vi "Do Zig Zag.vi"(9 "Wall Left?":bool=TRUE) -> (1 "Target Angle":dbl=1.5707963267948966)   [LabVIEW 2017]
uses:
  Globals/Zig Zag Global.vi
  Globals/Pose.vi
panel:
  in  "Forward Distance":dbl=200.0
  in  "Current Point":i32=4
  out "Initial Encoder Position":cluster{"X":dbl, "Y":dbl}={"X"=3425.411384902823, "Y"=-4669.166577156122}
  out "Initial Wall Distance":dbl=209.0
  out "Initial Wall Angle":dbl=1.5707963267948966
  in  "Target Angles&X Points":T1(array[cluster])=[{"Target Angle"=0.7, "Target X Point"=200.0}, {"Target Angle"=-0.7, "Target X Point"=280.0}, {"Target Angle"=0.5, "Target X Point"=250.0}]
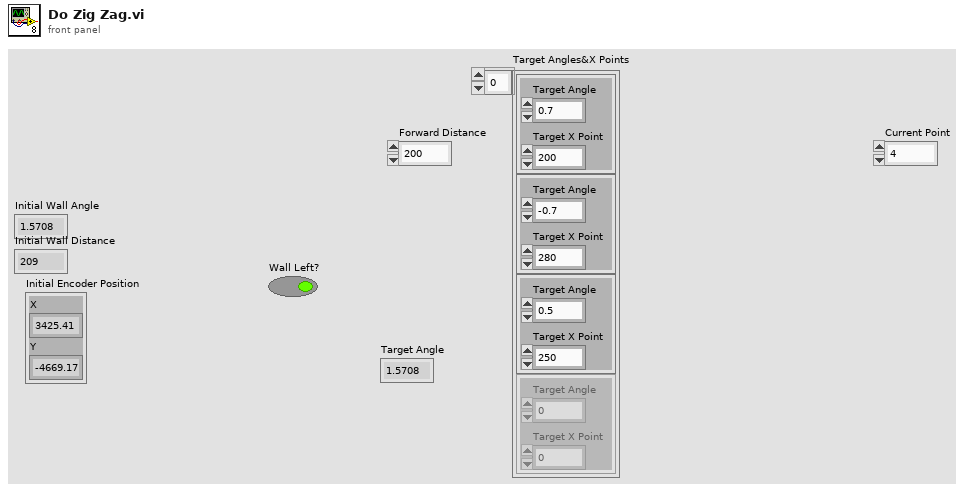
[diagram p1: front panel]
types:
  T1 = cluster{"Target Angle":dbl, "Target X Point":dbl}[]
  T2 = cluster{"Target Angle":dbl, "Target X Point":dbl}
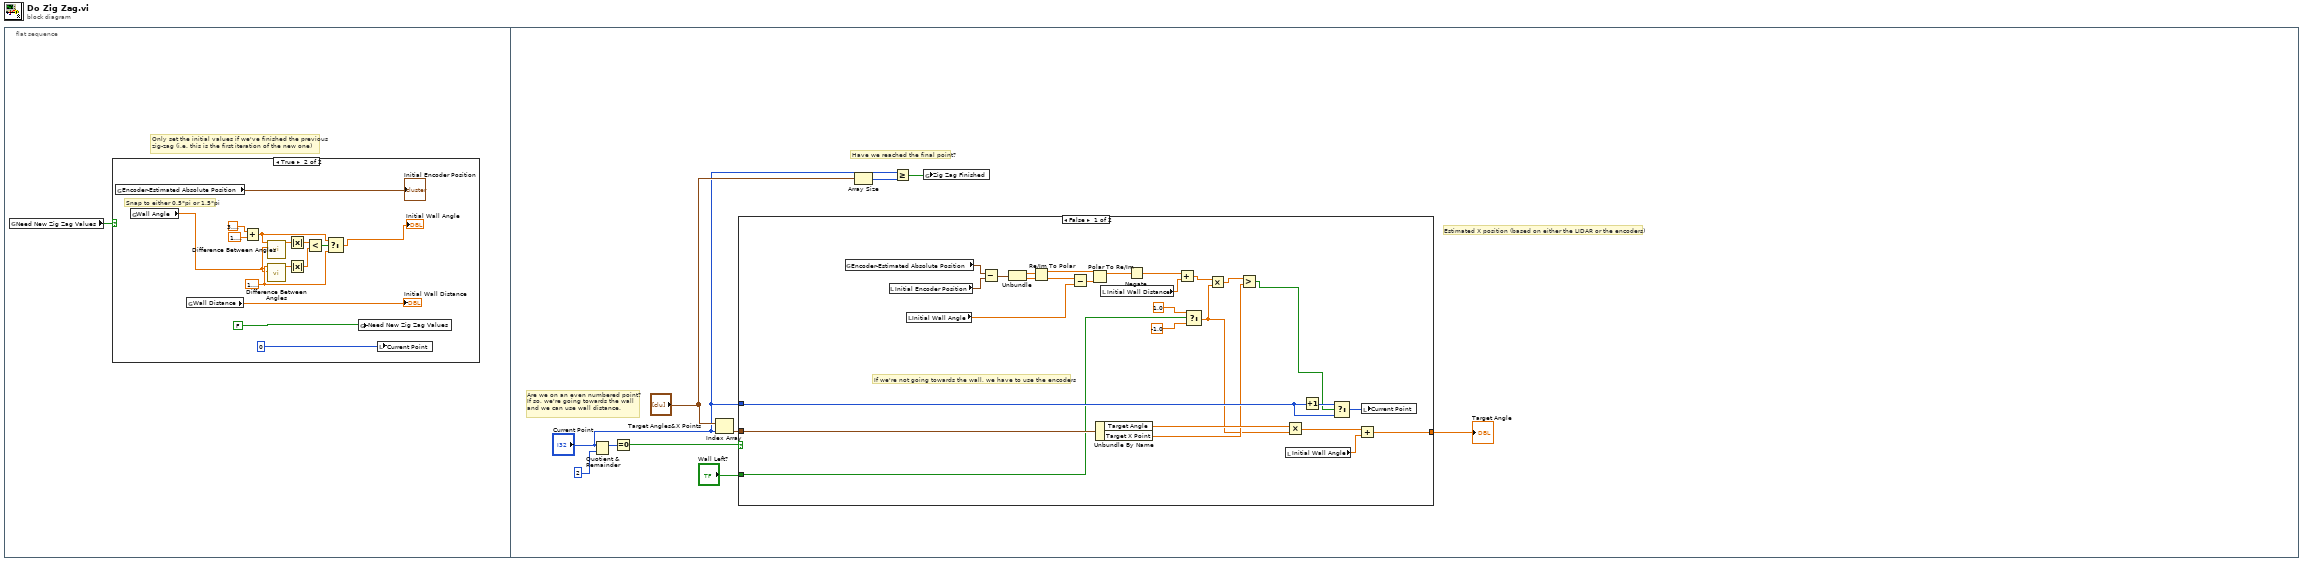
[diagram p0: block diagram]
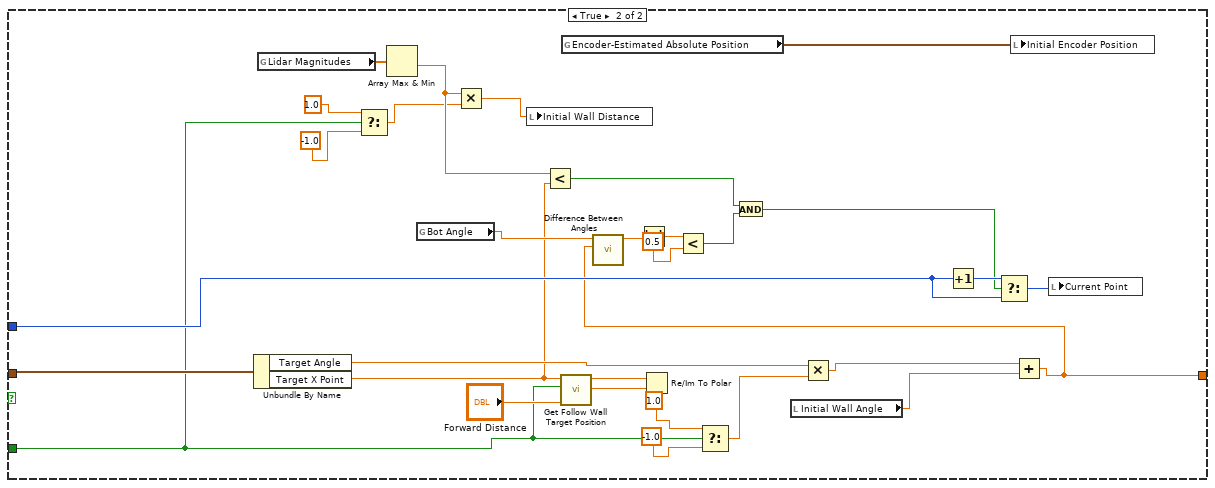
[diagram p3: hidden frame]
diagram:
  n1 = flat-sequence {
    frame #0 {
      # "Only set the initial values if we've finished the previous zig-zag (i.e. this is the first iteration of the new one)"
      n2 = global read "Zig Zag Global.vi" "Need New Zig Zag Values"() -> (w1:bool)
      n3 = case shown="True" w1 {
        frame False {
        }
        frame True {
          w4 = 1.5707963267948966
          # "Snap to either 0.5*pi or 1.5*pi"
          n4 = global read "Pose.vi" "Encoder-Estimated Absolute Position"() -> (→"Initial Encoder Position":cluster{"X":dbl, "Y":dbl})
          n5 = global read "Pose.vi" "Wall Angle"() -> (w2:dbl)
          n6 = global read "Pose.vi" "Wall Distance"() -> (→"Initial Wall Distance":dbl)
          n7 = Add(x=3.141592653589793, y=1.5707963267948966) -> (x+y=w5:dbl)
          n8 = call "Difference Between Angles.vi"("Angle 2"=w2, "Angle 1"=w5) -> ("Difference"=w10:dbl)  [unwired: 9 in]
          n9 = call "Difference Between Angles.vi"("Angle 2"=w2, "Angle 1"=w4) -> ("Difference"=w9:dbl)  [unwired: 9 in]
          n10 = Absolute Value(x=w10) -> (abs(x)=w7:dbl)
          n11 = Absolute Value(x=w9) -> (abs(x)=w6:dbl)
          n12 = Less?(x=w7, y=w6) -> (x < y?=w8:bool)
          n13 = Select(t=w5, s=w8, f=w4) -> (s? t:f=→"Initial Wall Angle":dbl)
          n14 = global write "Zig Zag Global.vi" "Need New Zig Zag Values"(FALSE ("Zig Zag Finished")) -> ()
          n15 = local write "Current Point"(0 ("Current Point")) -> ()
        }
      }
    }
    frame #1 {
      # "Estimated X position (based on either the LIDAR or the encoders)"
      # "Are we on an even numbered point?\nIf so, we're going towards the wall\nand we can use wall distance."
      # "Have we reached the final point?"
      n16 = Quotient & Remainder(x="Current Point", y=2) -> (x-y*floor(x/y)=w24:i32)  [unwired: 1 out]
      n17 = Equal To 0?(x=w24) -> (x = 0?=w23:bool)
      n18 = Index Array(array="Target Angles&X Points", index="Current Point") -> (element=w21:T2)
      n19 = case shown="False" w23 {
        tunnel: w21 -> [w40 w84]
        tunnel: "Wall Left?" -> [w33 w58]
        tunnel: [w32 w64] -> w17
        tunnel: "Current Point" -> [w35 w79]
        frame False {
          # "If we're not going towards the wall, we have to use the encoders"
          n20 = global read "Pose.vi" "Encoder-Estimated Absolute Position"() -> (w43:cluster{"X":dbl, "Y":dbl})
          n21 = local read "Initial Encoder Position"() -> (w52:cluster{"X":dbl, "Y":dbl})
          n22 = local read "Initial Wall Angle"() -> (w53:dbl)
          n23 = Subtract(x=w43, y=w52) -> (x-y=w51:cluster{"X":dbl, "Y":dbl})
          n24 = Unbundle(w51) -> ("X"=w50:dbl, "Y"=w49:dbl)
          n25 = Re/Im To Polar(2:w49, 3:w50) -> (0:w48:dbl, 1:w46:dbl)
          n26 = Subtract(x=w48, y=w53) -> (x-y=w47:dbl)
          n27 = Polar To Re/Im(2:w47, 3:w46) -> (1:w45:dbl)  [unwired: 1 out]
          n28 = Unbundle By Name(w40) -> ("Target Angle"=w34:dbl, "Target X Point"=w31:dbl)
          n29 = local read "Initial Wall Distance"() -> (w54:dbl)
          n30 = Negate(x=w45) -> (-x=w44:dbl)
          n31 = Add(x=w44, y=w54) -> (x+y=w29:dbl)
          n32 = Select(t=1.0, s=w33, f=-1.0) -> (s? t:f=w28:dbl)
          n33 = Multiply(x=w29, y=w28) -> (x*y=w27:dbl)
          n34 = Greater?(x=w27, y=w31) -> (0:w30:bool)
          n35 = local read "Initial Wall Angle"() -> (w39:dbl)
          n36 = Multiply(x=w34, y=w28) -> (x*y=w38:dbl)
          n37 = Increment(x=w35) -> (x+1=w36:i32)
          n38 = Select(t=w36, s=w30, f=w35) -> (s? t:f=w37:i32)
          n39 = Add(x=w38, y=w39) -> (x+y=w32:dbl)
          n40 = local write "Current Point"(w37) -> ()
        }
        frame True {
          n41 = Unbundle By Name(w84) -> ("Target Angle"=w65:dbl, "Target X Point"=w63:dbl)
          n42 = global read "Pose.vi" "Lidar Magnitudes"() -> (w61:dbl[])
          n43 = Select(t=1.0, s=w58, f=-1.0) -> (s? t:f=w56:dbl)
          n44 = Array Max & Min(array=w61) -> (min value=w57:dbl)  [unwired: 3 out]
          n45 = global read "Pose.vi" "Bot Angle"() -> (w66:dbl)
          n46 = Multiply(x=w57, y=w56) -> (x*y=w55:dbl)
          n47 = local write "Initial Wall Distance"(w55) -> ()
          n48 = Less?(x=w57, y=w63) -> (x < y?=w62:bool)
          n49 = call "Get Follow Wall Target Position.vi"("Forward Distance"="Forward Distance", "Wall left?"=w58, "Target Distance"=w63) -> ("Target Y (Relative)"=w82:dbl, "Target X (Relative)"=w83:dbl)  [unwired: 5 in]
          n50 = global read "Pose.vi" "Encoder-Estimated Absolute Position"() -> (w77:cluster{"X":dbl, "Y":dbl})
          n51 = Re/Im To Polar(2:w82, 3:w83) -> ()  [unwired: 2 out]
          n52 = Select(t=1.0, s=w58, f=-1.0) -> (s? t:f=w68:dbl)
          n53 = local read "Initial Wall Angle"() -> (w71:dbl)
          n54 = Multiply(x=w65, y=w68) -> (x*y=w69:dbl)
          n55 = Increment(x=w79) -> (x+1=w80:i32)
          n56 = local write "Initial Encoder Position"(w77) -> ()
          n57 = Add(x=w69, y=w71) -> (x+y=w64:dbl)
          n58 = call "Difference Between Angles.vi"("Angle 2"=w64, "Angle 1"=w66) -> ("Difference"=w76:dbl)  [unwired: 9 in]
          n59 = Absolute Value(x=w76) -> (abs(x)=w75:dbl)
          n60 = Less?(x=w75, y=0.5) -> (x < y?=w73:bool)
          n61 = And(x=w62, y=w73) -> (x .and. y?=w72:bool)
          n62 = Select(t=w80, s=w72, f=w79) -> (s? t:f=w81:i32)
          n63 = local write "Current Point"(w81) -> ()
        }
      }
      "Target Angle" <- w17
      n64 = Array Size(array="Target Angles&X Points") -> (size(s)=w26:i32)
      n65 = Greater Or Equal?(x="Current Point", y=w26) -> (x >= y?=w18:bool)
      n66 = global write "Zig Zag Global.vi" "Zig Zag Finished"(w18) -> ()
    }
  }
